vi "Offline_Analysis__SWLDA_분석기_woF4.vi"(0 "LDA_matrix":path caption="LDA_matrix.txt", 1 "DIscard Channel Info":i32[](array[numeric]), 5 "Weight":path caption="weight.txt", 7 "Target_order.txt":path, 9 "mius_flash_order":path, 11 "Brain":path, 12 "피험자이름":string, 13 "Save_path":string="ch\\ABM_Analysis\\ABM_Analysis_Data_150304\\OhJinHyuk_ABM_150305\\Test_Result\\") -> ()   [LabVIEW 2014]
uses:
  <vilib>/Utility/file.llb/Read From Spreadsheet File (DBL).vi
  <vilib>/Analysis/Matrix/Numeric/Conversions/Array To Matrix - RA2.vi
  <vilib>/Analysis/Matrix/Numeric/Conversions/Array To Matrix - RA.vi
  <vilib>/Utility/file.llb/Read From Spreadsheet File (I64).vi
  <vilib>/Utility/file.llb/Write To Spreadsheet File (DBL).vi
  <vilib>/Utility/file.llb/Write To Spreadsheet File (I64).vi
  <vilib>/Utility/file.llb/Write To Spreadsheet File (string).vi
  <vilib>/Analysis/Matrix/NI_Matrix.lvlib
panel:
  out "ACC":i16
  in  "Channel selection":bool[](array[boolean])=[TRUE, TRUE, TRUE, TRUE, TRUE, TRUE, TRUE, TRUE, TRUE, TRUE, TRUE]
  out "Target_order":i64[](array[numeric])
  out "Selected_Target":i32[](array[numeric])
  out "Accuracy":i16[](array[numeric])
  out "error out":errorcluster={"status"=TRUE, "code"=10, "source"="Create Folder in Offline_Analysis__SWLDA_분석기.vi->분석기_v2.vi<APPEND>\nC:\\Emotion_Research\\ABM_Analysis\\ABM_Analysis_Data_150304\\OhJinHyuk_ABM_150305\\Test_Result\\오진혁_SWLDA_LDA_pe005pr01"}
  in  "Random_num":i32=6
  in  "Flash_Repeat":i32=20
  in  "Frame_Length":i32=10
  in  "Sampling_Rate":dbl=250.0
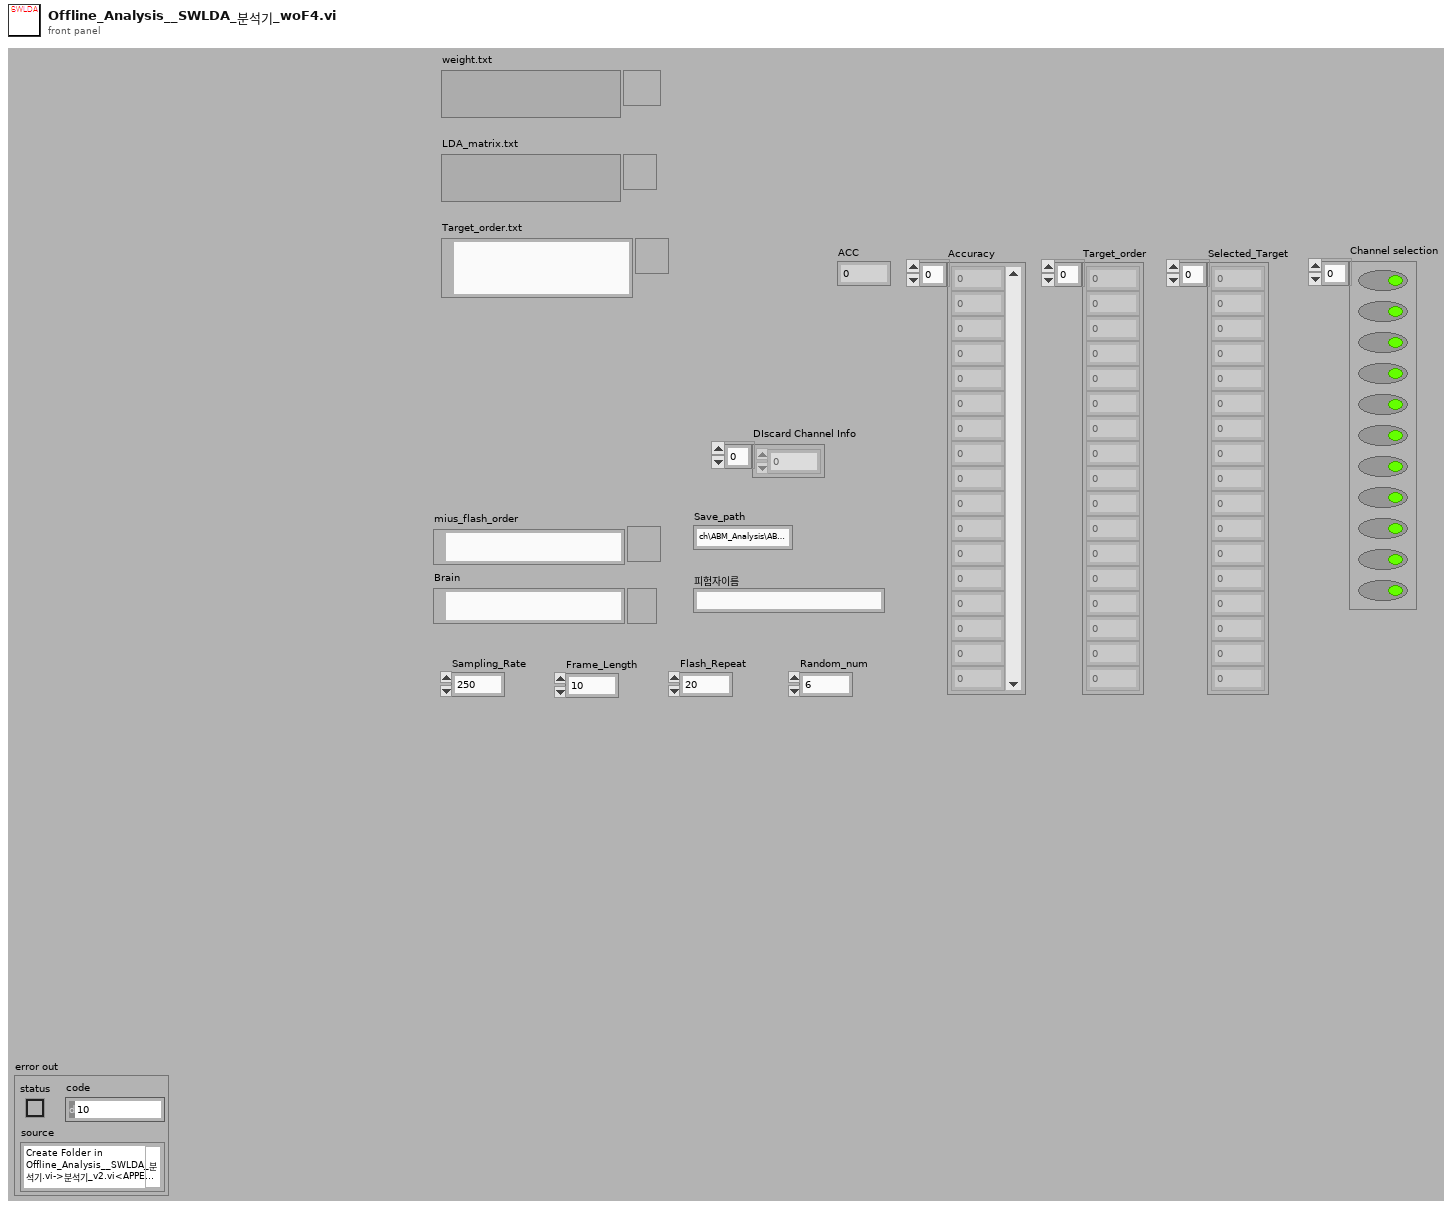
[diagram p1: front panel]
types:
  T1 = typedef "NI_Matrix.lvlib/RealMatrix.ctl" = dbl[][]
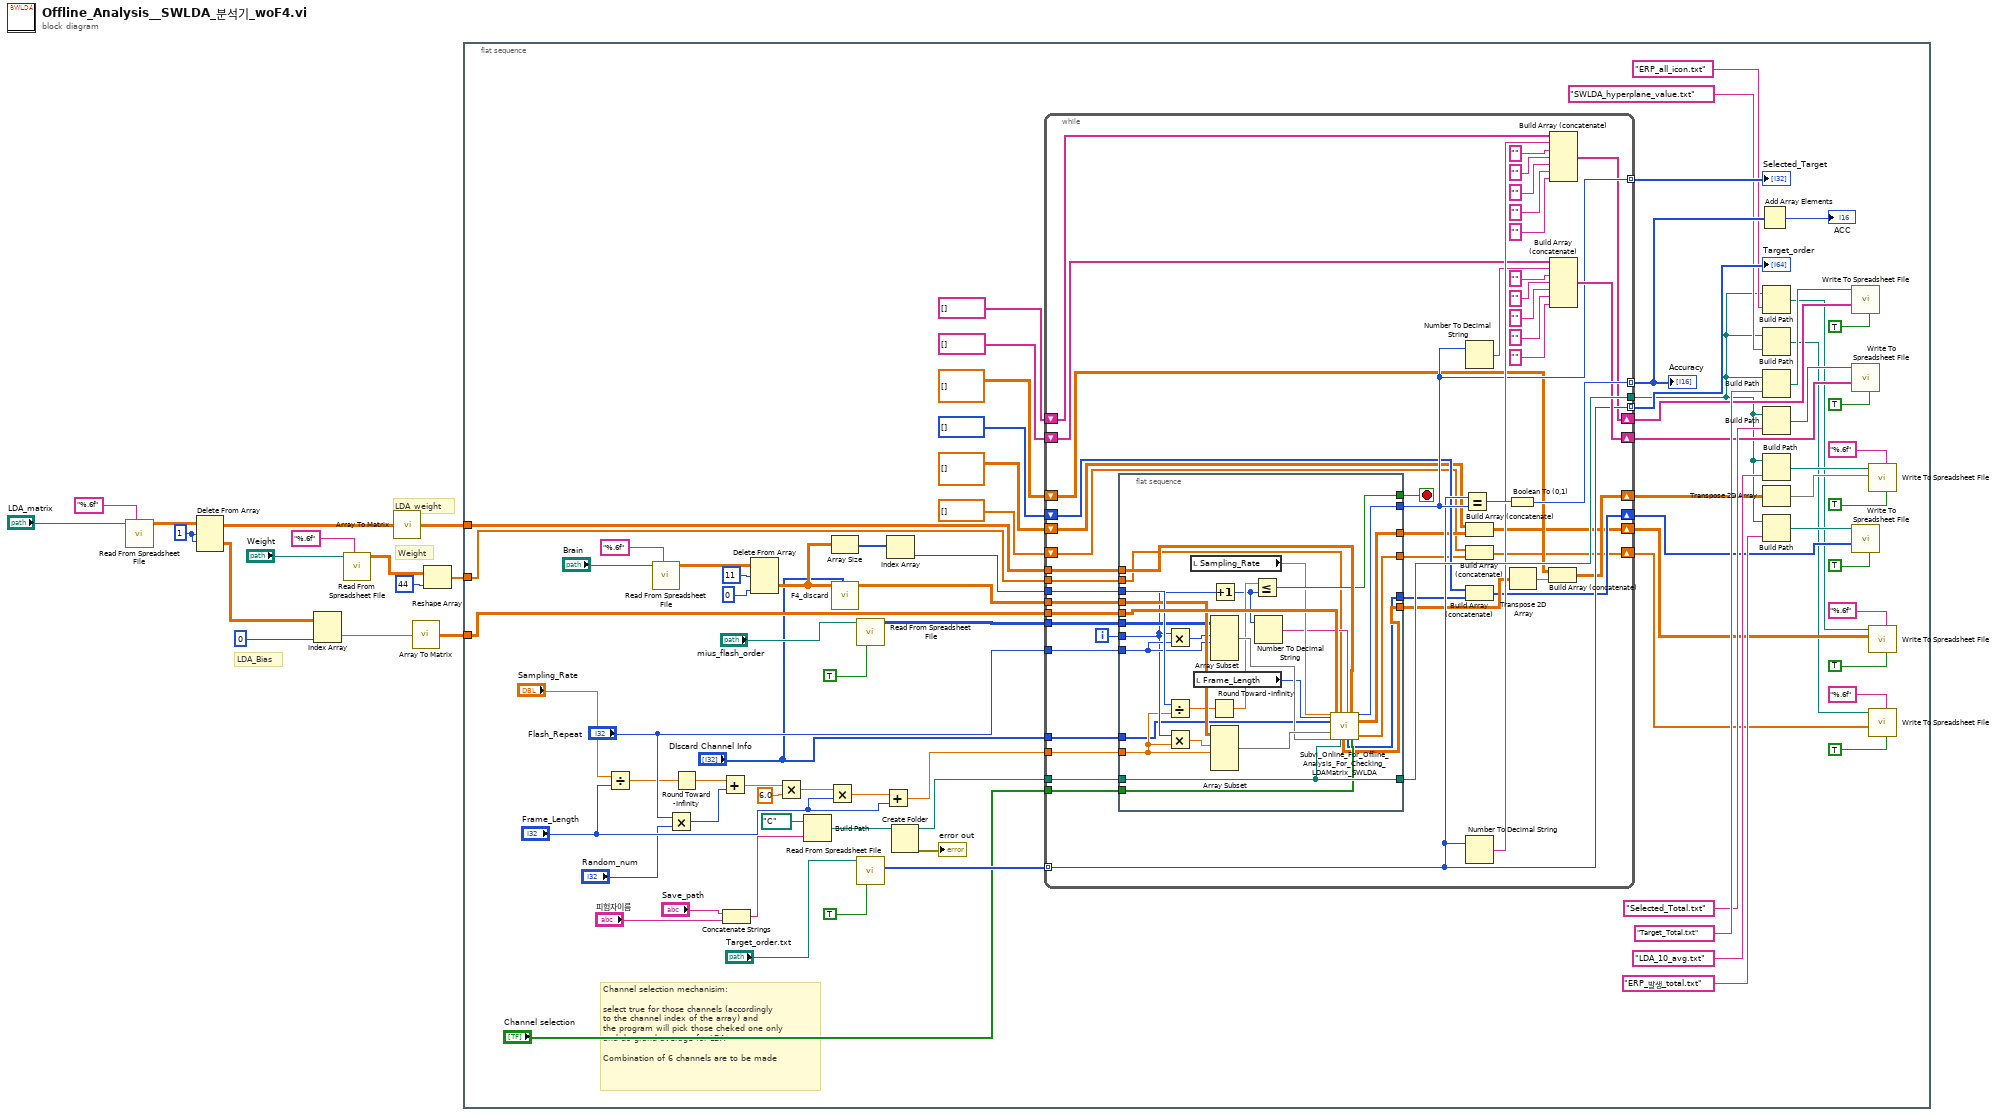
[diagram p0: block diagram]
diagram:
  w10 = 1 ("인덱스 (행)")
  # "LDA_Bias"
  # "LDA_weight"
  # "Weight"
  n1 = call-poly <vilib>:"Read From Spreadsheet File.vi"("format (%.3f)"="%.6f", "file path (dialog if empty)"="LDA_matrix") -> ("all rows"=w8:dbl[][])  [unwired: 5 in, 4 out]
  n2 = Delete From Array(array=w8, length=w10, index (row)=w10) -> (deleted portion=w13:dbl[][], array with subset deleted=w12:dbl[][])  [unwired: 1 in]
  n3 = Index Array(array=w13, index (col)=0 ("인덱스")) -> (element=w11:dbl[])  [unwired: 1 in]
  n4 = call-poly <vilib>:"Read From Spreadsheet File.vi"("format (%.3f)"="%.6f", "file path (dialog if empty)"="Weight") -> ("all rows"=w3:dbl[][])  [unwired: 5 in, 4 out]
  n5 = call-poly <vilib>:"Array To Matrix.vi"("Real 2D Array"=w12) -> ("Real Matrix"=w7:T1)
  n6 = call-poly <vilib>:"Array To Matrix.vi"("Real 1D Array"=w11) -> ("Real Matrix (Column Vector)"=w6:T1)
  n7 = Reshape Array(w3, 44 ("dimension size")) -> (w2:dbl[])
  n8 = flat-sequence {
    tunnel: w7 -> [w35]
    tunnel: w6 -> [w34]
    tunnel: w2 -> [w33]
    frame #0 {
      # "Channel selection mechanisim:\n\nselect true for those channels (accordingly\nto the channel index of the array) and \nthe program will pick those cheked one only\nand do grand average for LDA\n\nCombination of 6 channels are to be made"
      n9 = Divide(x="Sampling_Rate", y="Frame_Length") -> (x/y=w77:dbl)
      n10 = call-poly <vilib>:"Read From Spreadsheet File.vi"("format (%.3f)"="%.6f", "file path (dialog if empty)"="Brain") -> ("all rows"=w70:dbl[][])  [unwired: 5 in, 4 out]
      n11 = Multiply(x="Flash_Repeat", y="Random_num") -> (x*y=w80:i32)
      n12 = Round Toward -Infinity(1:w77) -> (0:w79:dbl)
      n13 = Add(x=w79, y=w80) -> (x+y=w82:dbl)
      n14 = Concatenate Strings("Save_path", "피험자이름") -> (w19:string)
      n15 = Delete From Array(array=w70, length=11 ("길이"), index (col)=0 ("비활성화된 인덱스 (열)")) -> (deleted portion=w73:dbl[][])  [unwired: 1 in, 1 out]
      n16 = Multiply(x=w82, y=6.0) -> (x*y=w84:dbl)
      n17 = Build Path(base path=path "C:/" ("path"), name or relative path=w19) -> (appended path=w89:path)
      n18 = Multiply(x=w84, y="Frame_Length") -> (x*y=w86:dbl)
      n19 = Array Size(array=w73) -> (size(s)=w74:i32[])
      n20 = call "F4_discard.vi"("DIscard Channel Info"="DIscard Channel Info", "Array"=w73) -> ("array w/ subset deleted"=w17:dbl[][])  [unwired: 9 in]
      n21 = call-poly <vilib>:"Read From Spreadsheet File.vi"("transpose (no:F)"=TRUE, "file path (dialog if empty)"="mius_flash_order") -> ("all rows"=w72:i64[][])  [unwired: 5 in, 4 out]
      n22 = call-poly <vilib>:"Read From Spreadsheet File.vi"("transpose (no:F)"=TRUE, "file path (dialog if empty)"="Target_order.txt") -> ("first row"=w64:i64[])  [unwired: 5 in, 4 out]
      n23 = Add(x=w86, y="Frame_Length") -> (x+y=w87:dbl)
      n24 = Index Array(array=w74) -> (element=w75:i32)  [unwired: 1 in]
      n25 = Create Folder(path (use dialog)=w89) -> (created path=w91:path, error out=→"error out":errorcluster)  [unwired: 2 in, 1 out]
      n26 = while {
        tunnel: w34 -> [w140]
        tunnel: w35 -> [w139]
        tunnel: w17 -> [w137]
        tunnel: w72 -> [w136]
        tunnel: w75 -> [w138]
        tunnel: w87 -> [w134]
        tunnel: "Flash_Repeat" -> [w135]
        tunnel: w91 -> [w133]
        tunnel: w64 -> [w111] mode=indexing
        tunnel: [w131] -> w55 mode=indexing
        tunnel: [w111] -> w61 mode=indexing
        tunnel: [w112] -> w62 mode=indexing
        tunnel: "Channel selection" -> [w128]
        tunnel: [w127] -> w20
        shift-right: [w114] -> w49
        shift-left: string[] [] -> [w113]
        shift-right: [w110] -> w48
        shift-left: string[] [] -> [w109]
        shift-right: [w106] -> w41
        shift-left: dbl[][] [] -> [w105]
        shift-right: [w103] -> w36
        shift-left: i16[] [] -> [w102]
        tunnel: w33 -> [w101]
        shift-right: [w100] -> w27
        shift-left: dbl[][] [] -> [w99]
        shift-right: [w96] -> w21
        shift-left: dbl[] [] -> [w95]
        tunnel: "DIscard Channel Info" -> [w94]
        i -> [w130]
        stop <- w129 stop-if-true
        n27 = flat-sequence {
          tunnel: [w168] -> w127
          tunnel: [w143] -> w98
          tunnel: w101 -> [w144]
          tunnel: [w145] -> w104
          tunnel: [w146] -> w107
          tunnel: w128 -> [w148]
          tunnel: [w149] -> w112
          tunnel: w133 -> [w168]
          tunnel: w134 -> [w155]
          tunnel: w130 -> [w156]
          tunnel: w135 -> [w158]
          tunnel: w136 -> [w160]
          tunnel: w137 -> [w163]
          tunnel: [w164] -> w129
          tunnel: w138 -> [w165]
          tunnel: w139 -> [w166]
          tunnel: w140 -> [w167]
          tunnel: [w142] -> w97
          tunnel: w94 -> [w141]
          frame #0 {
            n28 = Multiply(x=w156, y=w158) -> (x*y=w159:i32)
            n29 = Divide(x=w165, y=w155) -> (x/y=w154:dbl)
            n30 = Multiply(x=w156, y=w155) -> (x*y=w162:dbl)
            n31 = local read "Sampling_Rate"() -> (w152:dbl)
            n32 = local read "Frame_Length"() -> (w151:i32)
            n33 = Round Toward -Infinity(1:w154) -> (0:w153:dbl)
            n34 = Increment(x=w156) -> (x+1=w150:i32)
            n35 = Array Subset(array=w160, index (row)=w159, length (row)=w158) -> (w157:i64[][])  [unwired: 2 in]
            n36 = Array Subset(array=w163, index (row)=w162, length (row)=w155) -> (w161:dbl[][])  [unwired: 2 in]
            n37 = Less Or Equal?(x=w153, y=w150) -> (x <= y?=w164:bool)
            n38 = Number To Decimal String(number=w150) -> (decimal integer string=w147:string)  [unwired: 1 in]
            n39 = call "Subvi_Online_For_Offline_Analysis_For_Checking_LDAMatrix_SWLDA.vi"("rate"=w152, "samples per channel"=w151, "DIscard Channel Info"=w141, "Brain_data_source"=w161, "Target_Flash_Order"=w157, "Value"=w167, "Weight"=w144, "Path"=w168, "Number"=w147, "Matrix"=w166, "Channel selection"=w148) -> ("LDA_Parameter"=w146:dbl[][], "EPR_발생_total"=w145:i16[], "output-0~8"=w149:i32, "ERP_Parameters"=w143:dbl[][], "SWLDA"=w142:dbl[])  [unwired: 12 in]
          }
        }
        n40 = Equal?(x=w111, y=w112) -> (x = y?=w132:bool)
        n41 = Number To Decimal String(number=w112) -> (decimal integer string=w120:string)  [unwired: 1 in]
        n42 = Build Array (concatenate)(w99, w98) -> (w100:dbl[][])
        n43 = Build Array (concatenate)(w95, w97) -> (w96:dbl[])
        n44 = Build Array (concatenate)(w102, w104) -> (w103:i16[])
        n45 = Number To Decimal String(number=w111) -> (decimal integer string=w126:string)  [unwired: 1 in]
        n46 = Boolean To (0,1)(Boolean=w132) -> (0, 1=w131:i16)
        n47 = Transpose 2D Array(2D array=w107) -> (transposed array=w108:dbl[][])
        n48 = Build Array (concatenate)(w105, w108) -> (w106:dbl[][])
        n49 = Build Array (concatenate)(w109, w126, "" ("element"), "" ("element"), "" ("element"), "" ("element"), "" ("element")) -> (w110:string[])
        n50 = Build Array (concatenate)(w113, w120, "" ("element"), "" ("element"), "" ("element"), "" ("element"), "" ("element")) -> (w114:string[])
      }
      "Accuracy" <- w55
      "Selected_Target" <- w62
      "Target_order" <- w61
      n51 = Add Array Elements(numeric array=w55) -> (sum=→"ACC":i16)
      n52 = Build Path(base path=w20, name or relative path="ERP_all_icon.txt") -> (appended path=w30:path)
      n53 = Build Path(base path=w20, name or relative path="SWLDA_hyperplane_value.txt") -> (appended path=w22:path)
      n54 = Build Path(base path=w20, name or relative path="Target_Total.txt") -> (appended path=w57:path)
      n55 = Build Path(base path=w20, name or relative path="Selected_Total.txt") -> (appended path=w51:path)
      n56 = Build Path(base path=w20, name or relative path="LDA_10_avg.txt") -> (appended path=w44:path)
      n57 = Transpose 2D Array(2D array=w41) -> (transposed array=w42:dbl[][])
      n58 = Build Path(base path=w20, name or relative path="ERP_발생_total.txt") -> (appended path=w38:path)
      n59 = call-poly <vilib>:"Write To Spreadsheet File.vi"("transpose? (no:F)"=TRUE, "1D data"=w48, "file path (dialog if empty)"=w57) -> ()  [unwired: 5 in, 1 out]
      n60 = call-poly <vilib>:"Write To Spreadsheet File.vi"("transpose? (no:F)"=TRUE, "1D data"=w49, "file path (dialog if empty)"=w51) -> ()  [unwired: 5 in, 1 out]
      n61 = call-poly <vilib>:"Write To Spreadsheet File.vi"("transpose? (no:F)"=TRUE, "1D data"=w36, "file path (dialog if empty)"=w38) -> ()  [unwired: 5 in, 1 out]
      n62 = call-poly <vilib>:"Write To Spreadsheet File.vi"("transpose? (no:F)"=TRUE, "format (%.3f)"="%.6f", "2D data"=w42, "file path (dialog if empty)"=w44) -> ()  [unwired: 4 in, 1 out]
      n63 = call-poly <vilib>:"Write To Spreadsheet File.vi"("transpose? (no:F)"=TRUE, "format (%.3f)"="%.6f", "2D data"=w27, "file path (dialog if empty)"=w30) -> ()  [unwired: 4 in, 1 out]
      n64 = call-poly <vilib>:"Write To Spreadsheet File.vi"("transpose? (no:F)"=TRUE, "format (%.3f)"="%.6f", "1D data"=w21, "file path (dialog if empty)"=w22) -> ()  [unwired: 4 in, 1 out]
    }
  }
